vi "Create Tag Paths.vi"(7 "Create?":bool, 8 "error in (no error)":errorcluster, 10 "Names in":string[](array[string]), 11 "Process.Name":string) -> (0 "error out":errorcluster, 3 "Names out":string[](array[string]))   [LabVIEW 2019, in "Data Publishing Service.lvlib"]
uses:
  Data Publishing Service.lvlib
  <vilib>/Skyline/Utilities/Build Resource Name.vi
  <vilib>/Skyline/Tag/Shared/NI Skyline Tag.lvlib
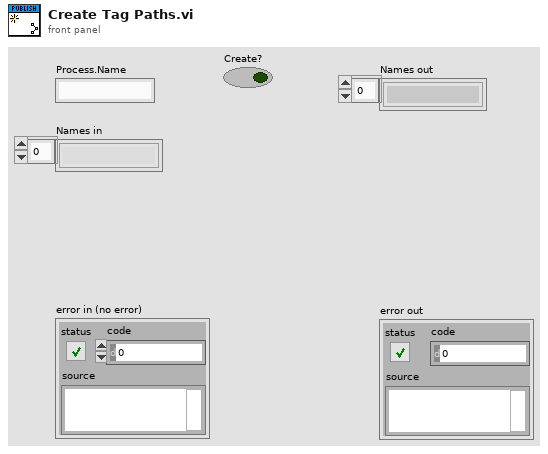
[diagram p1: front panel]
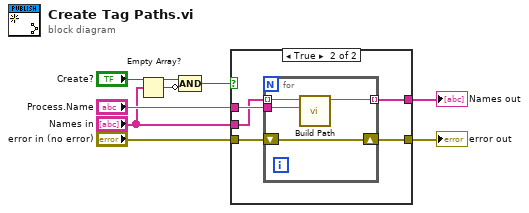
[diagram p0: block diagram]
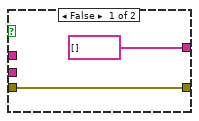
[diagram p2: hidden frame]
diagram:
  n1 = Empty Array?(array="Names in") -> (empty?=w2:bool)
  n2 = Compound Arithmetic op=AND("Create?", invert w2) -> (w3:bool)
  n3 = case shown="True" w3 {
    tunnel: "error in (no error)" -> [w10 w15]
    tunnel: "Process.Name" -> [_ w14]
    tunnel: [w10 w13] -> w7
    tunnel: "Names in" -> [_ w12]
    tunnel: [string[] [] ("Alias.Names") w11] -> w8
    frame False {
    }
    frame True {
      n4 = for {
        tunnel: w14 -> [w19]
        tunnel: w12 -> [w18] mode=indexing
        tunnel: [w16] -> w11 mode=indexing
        shift-right: [w17] -> w13
        shift-left: w15 -> [w17]
        n5 = call <vilib>:"Build Path.vi"("namespace"=w19, "tag name"=w18) -> ("path"=w16:string)  [unwired: 9 in]
      }
    }
  }
  "Names out" <- w8
  "error out" <- w7
